vi "PublicEval.vi"(8 "error in (no error)":errorcluster, 10 "Parents G":dbl, 11 "SudukuState in":refnum<class "SudukuState.lvclass">) -> (0 "error out":errorcluster, 1 "H":dbl, 2 "G":dbl, 3 "SudukuState out":refnum<class "SudukuState.lvclass">)   [LabVIEW 2009, in "SudukuState.lvclass"]
uses:
  SudukuState.lvclass
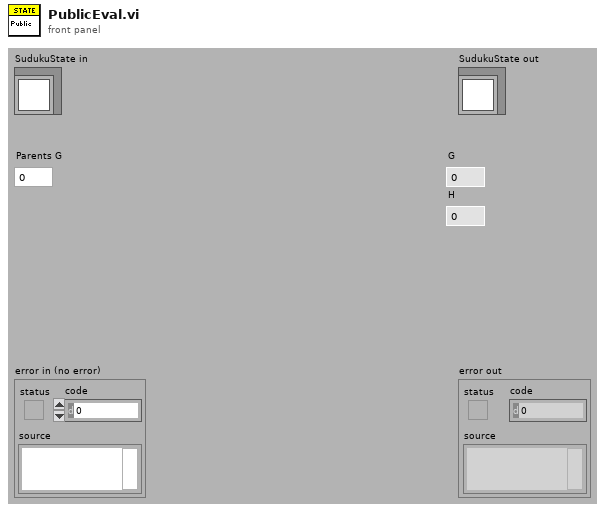
[diagram p1: front panel]
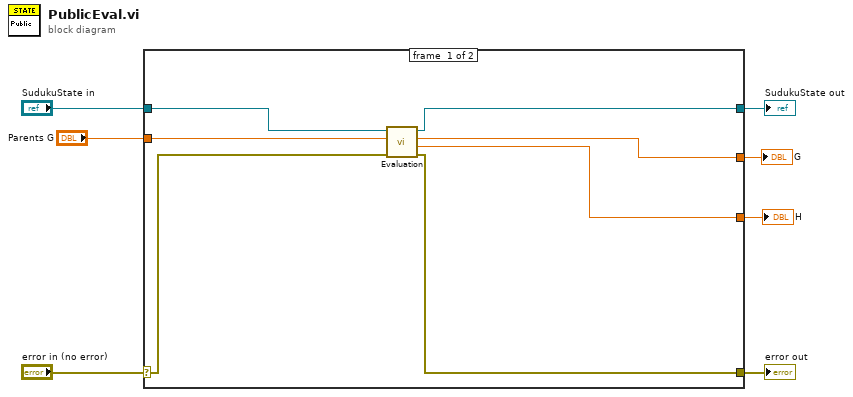
[diagram p0: block diagram]
diagram:
  n1 = case shown="Error" "error in (no error)" {
    selector: "error in (no error)" -> [w12 w16]
    tunnel: [w11 w16] -> w6
    tunnel: [w13 w15] -> w4
    tunnel: "SudukuState in" -> [w14 w15]
    tunnel: "Parents G" -> [w10 _]
    tunnel: [w9 _] -> w2
    tunnel: [w8 _] -> w1
    frame #0 {
      n2 = call-dynamic "Evaluation.vi"("error in (no error)"=w12, "Parents G"=w10, "SudukuState in"=w14) -> ("error out"=w11:errorcluster, "H"=w8:dbl, "G"=w9:dbl, "SudukuState out"=w13:refnum<class "SudukuState.lvclass">)  [unwired: 5 in]
    }
    frame #1 {
    }
  }
  "error out" <- w6
  "SudukuState out" <- w4
  "H" <- w1
  "G" <- w2
